vi "Add Record.vi"(8 "error in":errorcluster, 10 "Record":refnum<class "Record.lvclass">, 11 "Element in":refnum<class "Element.lvclass">) -> (0 "error out":errorcluster, 3 "Element out":refnum<class "Element.lvclass">)   [LabVIEW 2019, in "Element.lvclass"]
uses:
  Element.lvclass
  Record/Record.lvclass
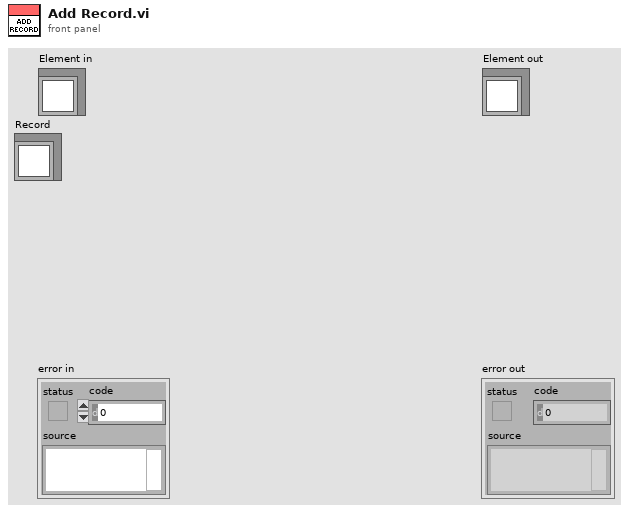
[diagram p1: front panel]
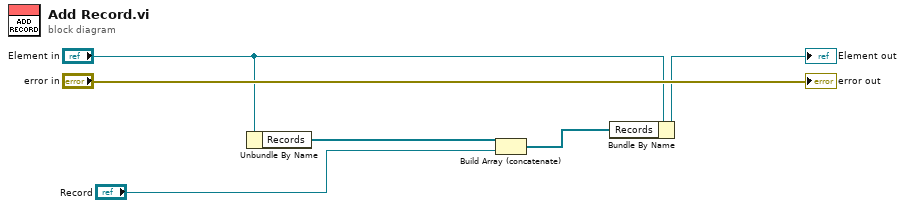
[diagram p0: block diagram]
diagram:
  n1 = Unbundle By Name("Element in") -> ("Records"=w3:refnum<class "Record.lvclass">[])
  n2 = Build Array (concatenate)(w3, "Record") -> (w2:refnum<class "Record.lvclass">[])
  n3 = Bundle By Name(cluster="Element in", "Records"=w2) -> (→"Element out":refnum<class "Element.lvclass">)
  "error out" <- "error in"
